vi "niRFUtil FWK Search String.vi"(7 "Delimiters":string[](array[string]), 8 "error in":errorcluster, 10 "Search String":string, 11 "Input String":string) -> (0 "error out":errorcluster, 1 "Whole Word Matched?":bool, 2 "Found String":string, 3 "Remaining String":string[](array[string]))   [LabVIEW 2015, in "niRFUtil.lvlib"]
uses:
  niRFUtil.lvlib
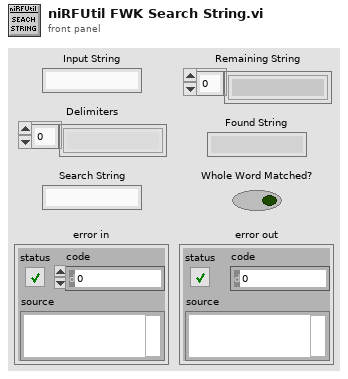
[diagram p1: front panel]
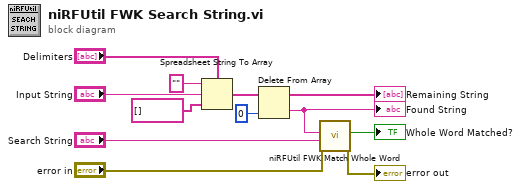
[diagram p0: block diagram]
diagram:
  n1 = Spreadsheet String To Array(delimiter (Tab)="Delimiters", format string="", spreadsheet string="Input String", array type (2D Dbl)=string[] [] ("Array in")) -> (array=w8:string[])
  n2 = Delete From Array(array=w8, index=0) -> (deleted portion=w9:string, array with subset deleted=→"Remaining String":string[])  [unwired: 1 in]
  "Found String" <- w9
  n3 = call "niRFUtil FWK Match Whole Word.vi"("error in"="error in", "Search String"="Search String", "Input String"=w9) -> ("error out"=→"error out":errorcluster, "Whole Word Matched?"=→"Whole Word Matched?":bool)  [unwired: 7 in]
